vi "Save DAC Configuration.vi"(8 "error in":errorcluster, 10 "Config File refnum in":T1, 11 "DAC Keller BNC in":refnum<class "DAC Keller BNC.lvclass">) -> (0 "error out":errorcluster, 2 "Config File refnum out":T1, 3 "DAC Keller BNC out":refnum<class "DAC Keller BNC.lvclass">)   [LabVIEW 2019, in "DAC.lvlib" / "DAC Keller BNC.lvclass"]
uses:
  DAC Keller BNC.lvclass
  C:/Users/wg/Documents/LV_Projects/test-stand/App/DAC/DAC.lvclass
  <vilib>/Utility/config.llb/Config Data RefNum.ctl
  DAC.lvclass/DAC.ctl
  DAC Keller BNC.lvclass/DAC Keller BNC.ctl
  DAC.lvclass
  <vilib>/Utility/config.llb/Write Key (String).vi
  <vilib>/Utility/config.llb/NI_LVConfig.lvlib
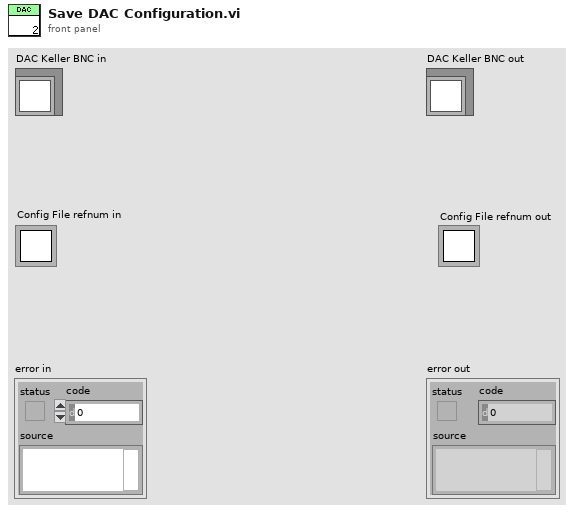
[diagram p1: front panel]
types:
  T1 = typedef "NI_LVConfig.lvlib/Config Data RefNum.ctl" = refnum<k1>
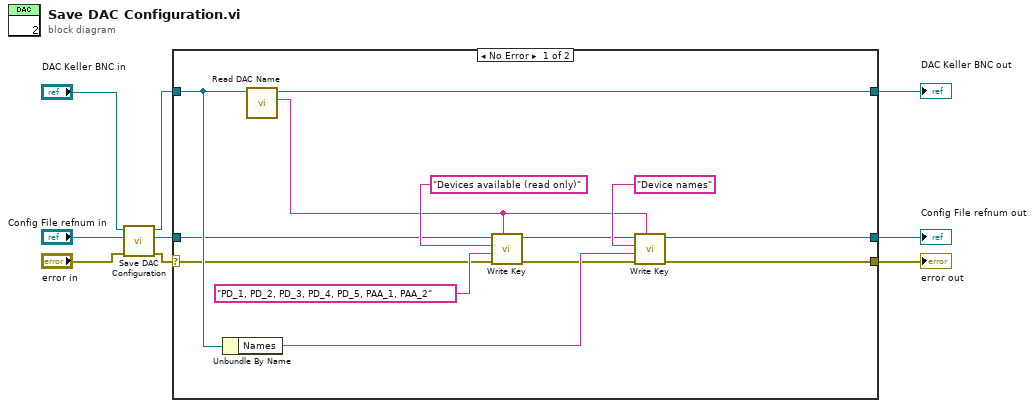
[diagram p0: block diagram]
diagram:
  n1 = call-parent "Save DAC Configuration.vi"("error in"="error in", "Config File refnum in"="Config File refnum in", "DAC in"="DAC Keller BNC in") -> ("error out"=w4:errorcluster, "Config File refnum out"=w5:T1, "DAC out"=w6:refnum<class "DAC Keller BNC.lvclass">)  [unwired: 6 in]
  n2 = case shown="No Error" w4 {
    selector: w4 -> [w12 w25]
    tunnel: [w17 w25] -> w1
    tunnel: [w20 w24] -> w3
    tunnel: w6 -> [w21 w24]
    tunnel: w5 -> [w11 w23]
    tunnel: [w18 w23] -> w2
    frame No Error {
      n3 = Unbundle By Name(w21) -> ("Names"=w19:string)
      n4 = call "Read DAC Name.vi"("DAC in"=w21) -> ("DAC Name"=w13:string, "DAC out"=w20:refnum<class "DAC Keller BNC.lvclass">)  [unwired: 8 in, 1 out]
      n5 = call-poly <vilib>:"Write Key.vi"("section"=w13, "error in (no error)"=w12, "value"="PD_1, PD_2, PD_3, PD_4, PD_5, PAA_1, PAA_2", "key"="Devices available (read only)", "refnum"=w11) -> ("error out"=w14:errorcluster, "refnum out"=w10:T1)  [unwired: 4 in, 1 out]
      n6 = call-poly <vilib>:"Write Key.vi"("section"=w13, "error in (no error)"=w14, "value"=w19, "key"="Device names", "refnum"=w10) -> ("error out"=w17:errorcluster, "refnum out"=w18:T1)  [unwired: 4 in, 1 out]
    }
    frame Error {
    }
  }
  "error out" <- w1
  "DAC Keller BNC out" <- w3
  "Config File refnum out" <- w2
